vi "calculate_hologram.vi"(7 "mainPos":T2, 8 "SLM1 cluster":T1={"1_Radio"=enum."Radio Selection 8", "1_Trans"=71.25748502994011, "1_Phase"=0.0, "1_HoloCode"="field = rho", "1_Semi"=FALSE, "1_Active"=0, "1_ModType"="_complex", "1_Flip"="no flip", "1_HoloNum"=87.0, "1_key1"="s", "1_value1"=-1, "1_key2"="m+1", "1_value2"=-1, "1_Calibration file"="IDSfirst_map_SLM1.pkl", "1_SLM brand"="SanTec"}, 10 "monoHolo in":T3=refnum, 11 "pySession":refnum<k35>) -> (3 "monoHolo out":T3)   [LabVIEW 2023]
uses:
  <vilib>/vision/Image Controls.llb/IMAQ Image.ctl
panel:
  in  "Numerical\nAperture":dbl=0.75
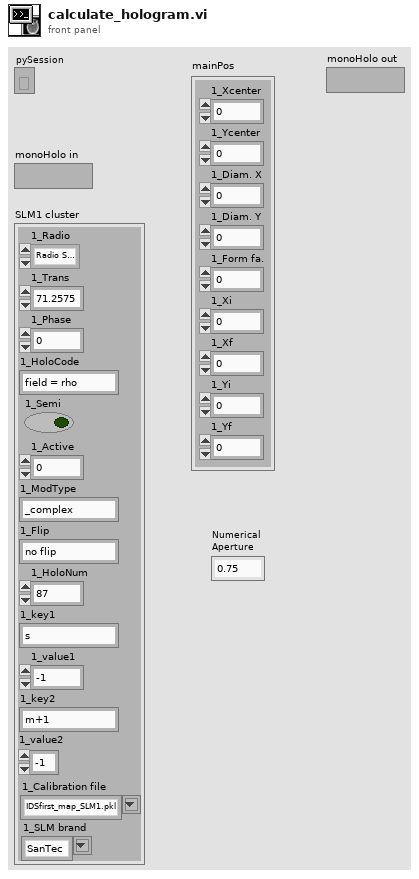
[diagram p1: front panel]
types:
  T1 = cluster{"1_Radio":enum32{"No Selection", "Radio Selection 1", "Radio Selection 2", "Radio Selection 3", "Radio Selection 4", "Radio Selection 5", "Radio Selection 6", "Radio Selection 7", "Radio Selection 8"}, "1_Trans":dbl, "1_Phase":dbl, "1_HoloCode":string, "1_Semi":bool, "1_Active":u16, "1_ModType":string, "1_Flip":string, "1_HoloNum":dbl, "1_key1":string, "1_value1":i64, "1_key2":string, "1_value2":i64, "1_Calibration file":string, "1_SLM brand":string}
  T2 = cluster{"1_Xcenter":dbl, "1_Ycenter":dbl, "1_Diam. X":dbl, "1_Diam. Y":dbl, "1_Form fa.":dbl, "1_Xi":dbl, "1_Xf":dbl, "1_Yi":dbl, "1_Yf":dbl}
  T3 = typedef "IMAQ Image.ctl" = refnum<image>
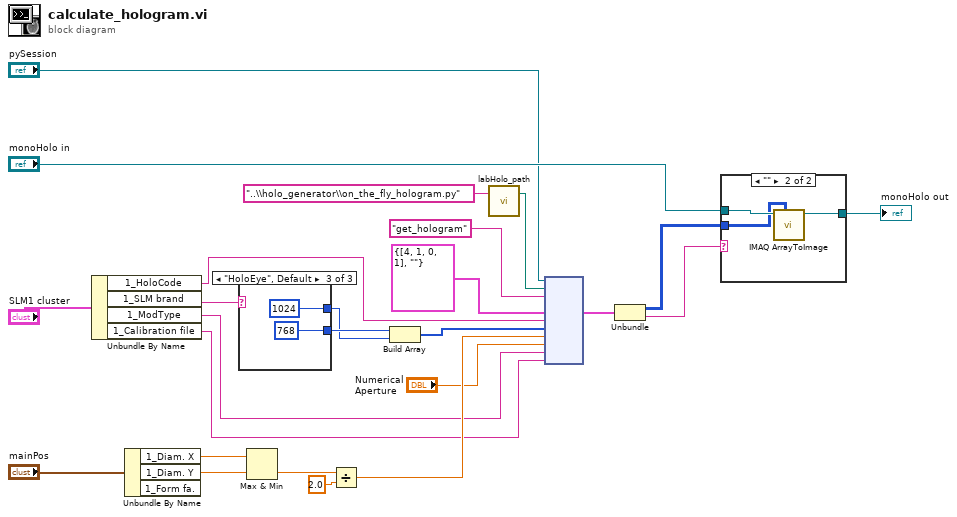
[diagram p0: block diagram]
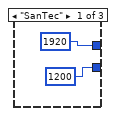
[diagram p2: hidden frame]
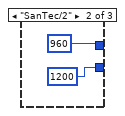
[diagram p3: hidden frame]
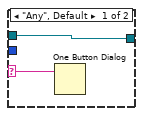
[diagram p4: hidden frame]
diagram:
  n1 = Unbundle By Name("SLM1 cluster") -> ("1_HoloCode"=w6:string, "1_SLM brand"=w10:string, "1_ModType"=w2:string, "1_Calibration file"=w1:string)
  n2 = Unbundle By Name("mainPos") -> ("1_Diam. X"=w15:dbl, "1_Diam. Y"=w14:dbl)  [unwired: 1 out]
  n3 = case shown="\"HoloEye\", Default" w10 {
    tunnel: [1200 1200 768] -> w9
    tunnel: [1920 960 1024] -> w8
    frame "SanTec" {
    }
    frame "SanTec/2" {
    }
    frame "HoloEye", Default {
    }
  }
  n4 = Max & Min(x=w15, y=w14) -> (min(x,y)=w13:dbl)  [unwired: 1 out]
  n5 = Divide(x=w13, y=2.0) -> (x/y=w4:dbl)
  n6 = Build Array(w9, w8) -> (w5:i32[])
  n7 = call "labHolo_path.vi"("sub folder or file (str)"="..\\holo_generator\\on_the_fly_hologram.py") -> ("labHolo path"=w17:path)  [unwired: 1 in, 1 out]
  n8 = node("pySession", w17, "get_hologram" ("function name"), cluster{u16[][], string} {[[4, 1], [0, 1]], ""}, w6, w5, w4, "Numerical\nAperture", w2, w1) -> (w23:cluster{u16[][], string})  [unwired: 7 in, 4 out]
  n9 = Unbundle(w23) -> (w24:u16[][], w25:string)
  n10 = case shown="\"\"" w25 {
    selector: w25 -> [w32 _]
    tunnel: "monoHolo in" -> [w33 w36]
    tunnel: [w33 w35] -> w19
    tunnel: w24 -> [_ w34]
    frame "Any", Default {
      n11 = One Button Dialog(message=w32) -> ()  [unwired: 1 in, 1 out]
    }
    frame "" {
      n12 = call "IMAQ ArrayToImage"("Image Pixels (U16)"=w34, "Image"=w36) -> ("Image Out"=w35:T3)  [unwired: 8 in, 1 out]
    }
  }
  "monoHolo out" <- w19
